vi "Connect.vi"(8 "error in (no error)":errorcluster) -> (0 "error out":errorcluster, 3 "function return":bool)   [LabVIEW 2013, in "PCTx.lvlib"]
doc: "DECLDIR bool Connect(void);"
uses:
  PCTx.lvlib
  PCTx.dll
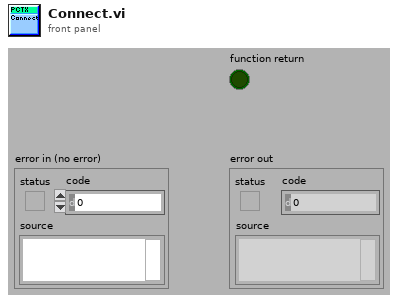
[diagram p1: front panel]
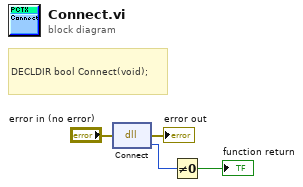
[diagram p0: block diagram]
diagram:
  # "DECLDIR bool Connect(void);"
  n1 = dll-call lib="C:/Users/user/Documents/Dropbox/Kettering/Robotics Team/RC Car Race Information/Teleop Labview Code/Winter '14 Force Feedback Experiment/PCTx Files/PCTx/PCTx.*" fn="Connect"(error in="error in (no error)") -> (error out=→"error out":errorcluster, w3:u8)  [unwired: 2 in, 1 out]
  n2 = Not Equal To 0?(x=w3) -> (x != 0?=→"function return":bool)
